vi "BPSK_MRX.vi"() -> ()   [LabVIEW 2012]
panel:
  in  "Carrier":dbl(slide) scale=0.0..5000.0
  in  "Binary Data":dbl(slide) scale=0.0..500.0
  out "Waveform Graph 3":dynamicdata(graph)
  out "Binary Data":dynamicdata(graph)
  out "BPSK":dynamicdata(graph)
  out "Demodulated PSK":dynamicdata(graph)
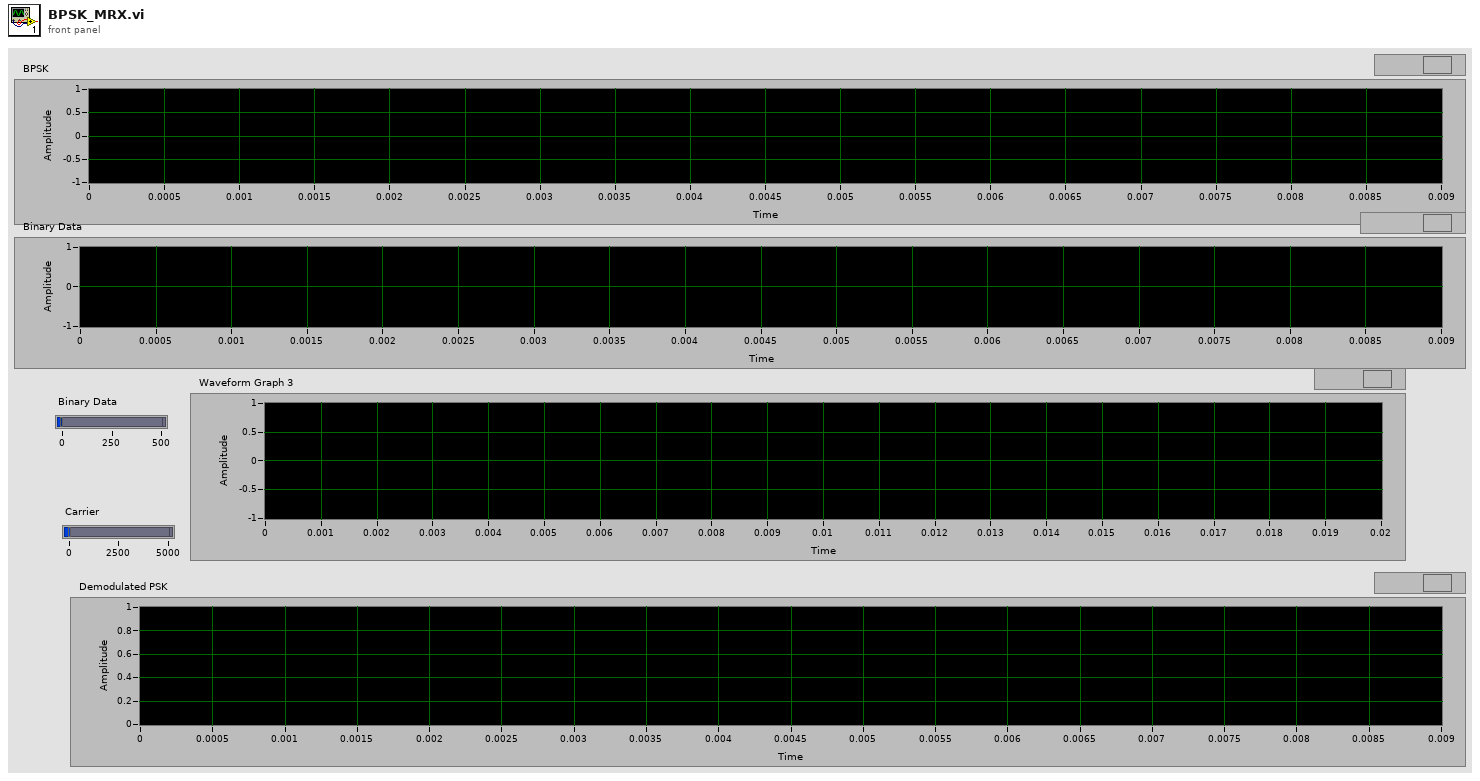
[diagram p1: front panel]
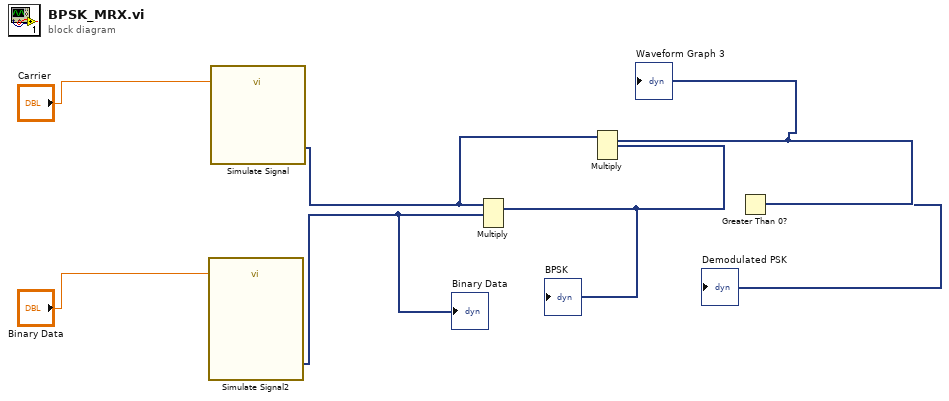
[diagram p0: block diagram]
diagram:
  n1 = call "Simulate Signal2"("Frequency"="Binary Data") -> ("Square"=w6:dynamicdata)  [unwired: 13 in, 1 out]
  "Binary Data" <- w6
  n2 = call "Simulate Signal"("Frequency"="Carrier") -> ("Sine"=w7:dynamicdata)  [unwired: 13 in, 1 out]
  n3 = Multiply(1:w6, 2:w7) -> (0:w5:dynamicdata)  [unwired: 1 in, 1 out]
  "BPSK" <- w5
  n4 = Multiply(1:w5, 2:w7) -> (0:w4:dynamicdata)  [unwired: 1 in, 1 out]
  "Waveform Graph 3" <- w4
  n5 = Greater Than 0?(x=w4) -> (x > 0?=→"Demodulated PSK":dynamicdata)
